vi "Gaussian Fit Guess Parameters.vi"(10 "Y Array":dbl[](array[numeric]), 11 "X Array":dbl[](array[numeric])) -> (3 "Gaussian Fit Parameters":T1)   [LabVIEW 2021, in "Fits.lvlib"]
uses:
  Gaussian Fit Parameters.ctl
  Fits.lvlib
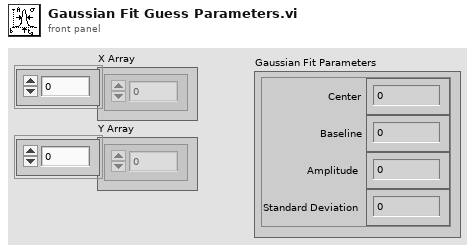
[diagram p1: front panel]
types:
  T1 = typedef "Fits.lvlib/Gaussian Fit Parameters.ctl" = cluster{"Center":dbl, "Baseline":dbl, "Amplitude":dbl, "Standard Deviation":dbl}
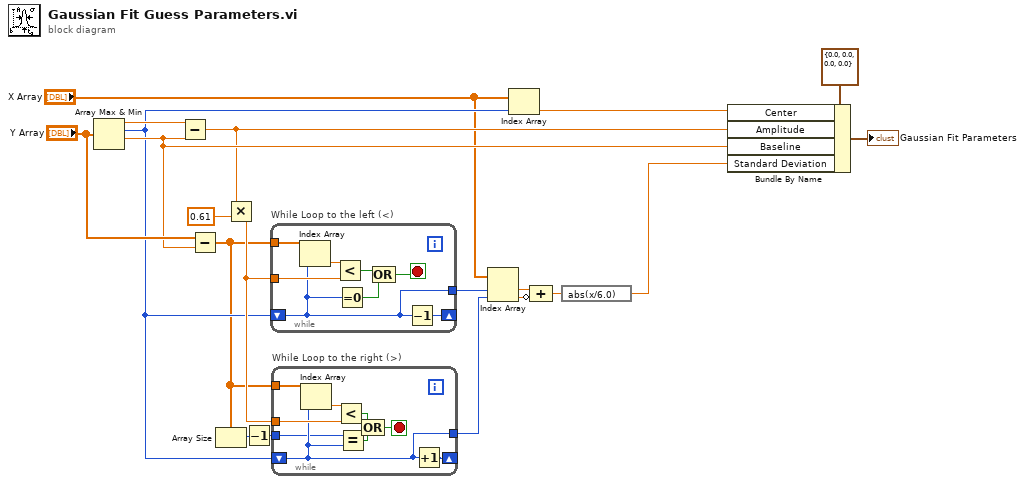
[diagram p0: block diagram]
diagram:
  n1 = Array Max & Min(array="Y Array") -> (max value=w20:dbl, max index (indices)=w13:i32, min value=w17:dbl)  [unwired: 1 out]
  n2 = Subtract(x=w20, y=w17) -> (x-y=w16:dbl)
  n3 = Subtract(x="Y Array", y=w17) -> (x-y=w12:dbl[])
  n4 = Array Size(array=w12) -> (size(s)=w11:i32)
  n5 = Multiply(x=w16, y=0.61) -> (x*y=w14:dbl)
  n6 = Decrement(x=w11) -> (x-1=w10:i32)
  n7 = while "While Loop to the left (<)" {
    shift-right: [w24] -> _
    shift-left: w13 -> [w21]
    tunnel: w12 -> [w28]
    tunnel: w14 -> [w26]
    tunnel: [w21] -> w8
    stop <- w23 stop-if-true
    n8 = Index Array(array=w28, index=w21) -> (element=w27:dbl)
    n9 = Less?(x=w27, y=w26) -> (x < y?=w25:bool)
    n10 = Equal To 0?(x=w21) -> (x = 0?=w22:bool)
    n11 = Compound Arithmetic op=OR(w25, w22) -> (w23:bool)
    n12 = Decrement(x=w21) -> (x-1=w24:i32)
  }
  n13 = while "While Loop to the right (>)" {
    shift-right: [w33] -> _
    shift-left: w13 -> [w30]
    tunnel: w12 -> [w37]
    tunnel: w14 -> [w35]
    tunnel: [w30] -> w7
    tunnel: w10 -> [w29]
    stop <- w32 stop-if-true
    n14 = Index Array(array=w37, index=w30) -> (element=w36:dbl)
    n15 = Less?(x=w36, y=w35) -> (x < y?=w34:bool)
    n16 = Equal?(x=w29, y=w30) -> (x = y?=w31:bool)
    n17 = Compound Arithmetic op=OR(w34, w31) -> (w32:bool)
    n18 = Increment(x=w30) -> (x+1=w33:i32)
  }
  n19 = Index Array(array="X Array", index #1=w8, index #2=w7) -> (element #1=w6:dbl, element #2=w5:dbl)
  n20 = Index Array(array="X Array", index=w13) -> (element=w19:dbl)
  n21 = Compound Arithmetic op=ADD(w6, invert w5) -> (w4:dbl)
  n22 = expression code="abs(x/6.0)"(w4) -> (w3:dbl)
  n23 = Bundle By Name(cluster=T1 {"Center"=0.0, "Baseline"=0.0, "Amplitude"=0.0, "Standard Deviation"=0.0} ("Gaussian Fit Parameters"), "Center"=w19, "Amplitude"=w16, "Baseline"=w17, "Standard Deviation"=w3) -> (→"Gaussian Fit Parameters":T1)
